vi "ZIDevice_GetDeviceSN.vi"(8 "error in (no error)":errorcluster, 10 "alias":string, 11 "Hardware Handle.Device Name":string[][](array[string])) -> (0 "error out":errorcluster, 2 "Device SN":string)   [LabVIEW 2016, in "General.lvlib"]
uses:
  General.lvlib
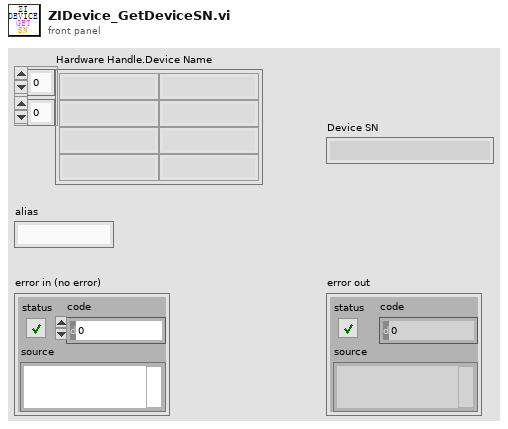
[diagram p1: front panel]
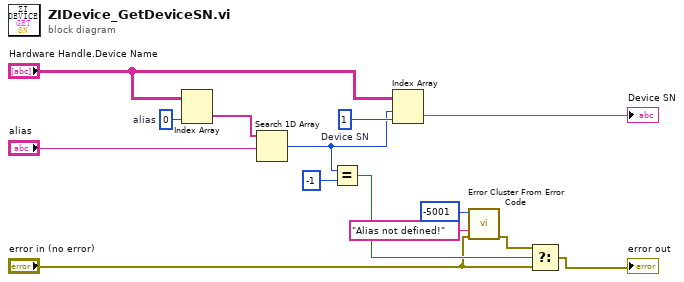
[diagram p0: block diagram]
diagram:
  w11 = 1  # Device SN
  w14 = 0  # alias
  n1 = Index Array(array="Hardware Handle.Device Name", index (col)=w14) -> (element=w13:string[])  [unwired: 1 in]
  n2 = Search 1D Array(1D array=w13, element="alias") -> (index of element=w8:i32)  [unwired: 1 in]
  n3 = Equal?(x=w8, y=-1) -> (x = y?=w6:bool)
  n4 = Index Array(array="Hardware Handle.Device Name", index (row)=w8, index (col)=w11) -> (element=→"Device SN":string)
  n5 = call <vilib>:"Error Cluster From Error Code.vi"("error in (no error)"="error in (no error)", "error message (\"\")"="Alias not defined!" ("error message (\"\")"), "error code (0)"=-5001 ("[error code] (0)")) -> ("error out"=w4:errorcluster)  [unwired: 6 in]
  n6 = Select(t=w4, s=w6, f="error in (no error)") -> (s? t:f=→"error out":errorcluster)
